vi "Set Class Instance.vi"(11 "OSC Type":string) -> (3 "element":refnum<class "Osciloscopio.lvclass">)   [LabVIEW 2020, in "Oscilloscope.lvlib"]
uses:
  Oscilloscope.lvlib
  Clases/Osciloscopio/Osciloscopio.lvclass
  Clases/TDS 2000/TDS 2000.lvclass
  C:/Users/ronad/Osciloscopio/Osciloscopio DQMH/Libraries/Oscilloscope/Clases/Osciloscopio/Osciloscopio.lvclass
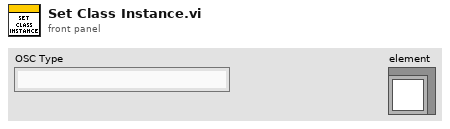
[diagram p1: front panel]
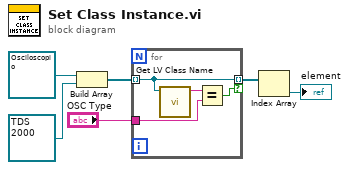
[diagram p0: block diagram]
diagram:
  n1 = Build Array(refnum<class "Osciloscopio.lvclass"> refnum ("Oscilloscope.lvlib:Osciloscopio.lvclass"), refnum<class "TDS 2000.lvclass"> refnum ("Oscilloscope.lvlib:TDS 2000.lvclass")) -> (w4:refnum<class "Osciloscopio.lvclass">[])
  n2 = for {
    tunnel: w4 -> [w10] mode=indexing
    tunnel: [w10] -> w3 mode=indexing if=w7
    tunnel: "OSC Type" -> [w8]
    n3 = call <vilib>:"Get LV Class Name.vi"("object"=w10) -> ("class name"=w9:string)  [unwired: 9 in, 1 out]
    n4 = Equal?(x=w9, y=w8) -> (x = y?=w7:bool)
  }
  n5 = Index Array(array=w3) -> (element=→"element":refnum<class "Osciloscopio.lvclass">)  [unwired: 1 in]
